vi "BMark_Change Bookmark Image.vi"(7 "Picture Control Reference":refnum<vi>, 8 "error in (no error)":errorcluster, 9 "No Image?":bool, 10 "bookmarks":T1[](array[typedef]), 11 "tag":string) -> (0 "error out":errorcluster)   [LabVIEW 2017]
uses:
  controls/BMark_Bookmark Data.ctl
  controls/BMark_VI_Identifier.ctl
  <vilib>/addons/analyzer/_analyzerctrls.llb/VIAnCtl Analysis App Info.ctl
  <vilib>/Utility/miscctls.llb/LVPointTypeDef.ctl
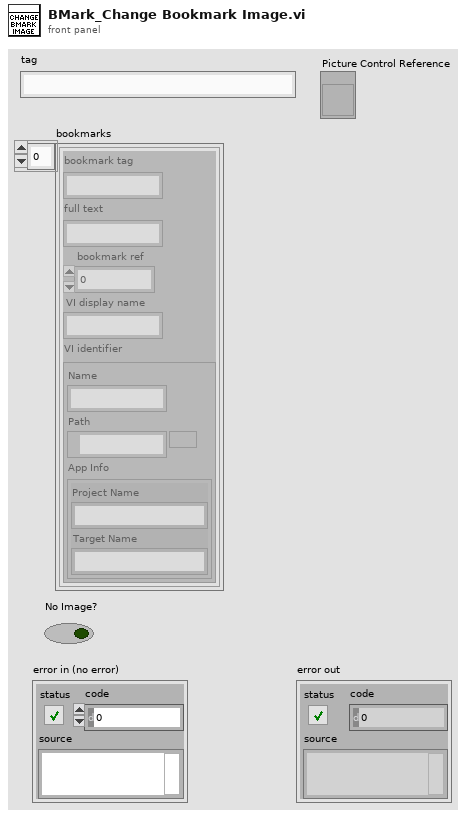
[diagram p1: front panel]
types:
  T1 = typedef "BMark_Bookmark Data.ctl" = cluster{"bookmark tag":string, "full text":string, "bookmark ref":i32, "VI display name":string, "VI identifier":T2}
  T2 = typedef "BMark_VI_Identifier.ctl" = cluster{"Name":string, "Path":path, "App Info":T3}
  T3 = typedef "VIAnCtl Analysis App Info.ctl" = cluster{"Project Name":string, "Target Name":string}
  T4 = typedef "LVPointTypeDef.ctl" = cluster{"Horizontal":i16, "Vertical":i16}
  T5 = cluster{"horizontal":enum16{"left", "center", "right"}, "vertical":enum16{"top", "center", "bottom"}}
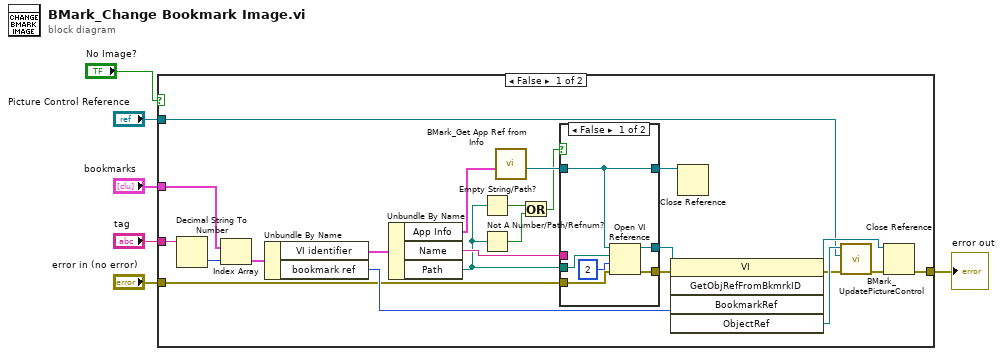
[diagram p0: block diagram]
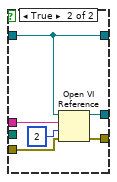
[diagram p2: hidden frame]
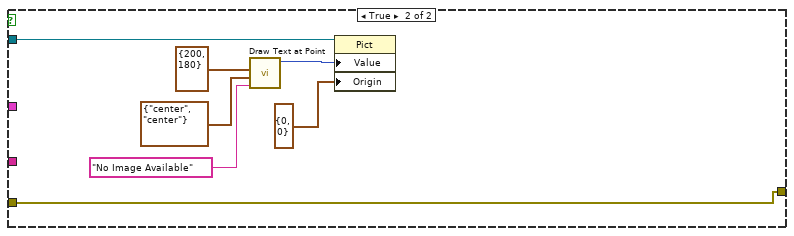
[diagram p3: hidden frame]
diagram:
  n1 = case shown="False" "No Image?" {
    tunnel: "tag" -> [w29 _]
    tunnel: "bookmarks" -> [w28 _]
    tunnel: [w22 w45] -> w4
    tunnel: "error in (no error)" -> [w11 w45]
    tunnel: "Picture Control Reference" -> [w9 w42]
    frame False {
      n2 = Decimal String To Number(string=w29) -> (number=w27:i32)  [unwired: 2 in, 1 out]
      n3 = Index Array(array=w28, index=w27) -> (element=w26:T1)
      n4 = Unbundle By Name(w26) -> ("VI identifier"=w25:T2, "bookmark ref"=w23:i32)
      n5 = Unbundle By Name(w25) -> ("App Info"=w20:T3, "Name"=w24:string, "Path"=w18:path)
      n6 = Empty String/Path?(string/path=w18) -> (empty?=w17:bool)
      n7 = Not A Number/Path/Refnum?(number/path/refnum=w18) -> (NaN/Path/Refnum?=w16:bool)
      n8 = call "BMark_Get App Ref from Info.vi"("Analysis App Info"=w20) -> ("Analysis App ref"=w19:refnum<vi>)  [unwired: 9 in, 1 out]
      n9 = Or(x=w17, y=w16) -> (x .or. y?=w15:bool)
      n10 = case shown="False" w15 {
        tunnel: w24 -> [_ w41]
        tunnel: w19 -> [w30 w36]
        tunnel: [w35 w40] -> w13
        tunnel: w18 -> [w34 _]
        tunnel: w11 -> [w33 w39]
        tunnel: [w32 w38] -> w14
        tunnel: [w30 w36] -> w21
        frame False {
          n11 = Open VI Reference(application reference (local)=w30, vi path=w34, options=2, error in (no error)=w33) -> (vi reference=w35:refnum<vi>, error out=w32:errorcluster)  [unwired: 2 in]
        }
        frame True {
          n12 = Open VI Reference(application reference (local)=w36, vi path=w41, options=2, error in (no error)=w39) -> (vi reference=w40:refnum<vi>, error out=w38:errorcluster)  [unwired: 2 in]
        }
      }
      n13 = invoke class="VI" method="GetObjRefFromBkmrkID"(reference=w13, error in=w14, "BookmarkRef"=w23) -> (reference out=w12:refnum<vi>, error out=w7:errorcluster, "ObjectRef"=w10:refnum<vi>)  [unwired: 2 in, 2 out]
      n14 = Close Reference(reference=w21) -> ()  [unwired: 1 in, 1 out]
      n15 = call "BMark_UpdatePictureControl.vi"("error in (no error)"=w7, "Picture Control Reference"=w9, "Center Object Reference"=w10) -> ("error out"=w8:errorcluster)  [unwired: 8 in]
      n16 = Close Reference(reference=w12, error in (no error)=w8) -> (error out=w22:errorcluster)
    }
    frame True {
      n17 = call <vilib>:"Draw Text at Point.vi"("text"="No Image Available", "alignment(left, top)"=T5 {"horizontal"=enum."center", "vertical"=enum."center"}, "origin"=cluster{"x":i16, "y":i16} {"x"=200, "y"=180}) -> ("new picture"=w44:picture)  [unwired: 7 in, 1 out]
      n18 = property class="Pict"(reference=w42, "Value"=w44, "Origin"=T4 {"Horizontal"=0, "Vertical"=0}) -> ()  [unwired: 1 in, 2 out]
    }
  }
  "error out" <- w4
